vi "SHT41-string-array-to-data.vi"(9 "Starting Index":i32, 11 "Data In (string array)":string[](array[string])) -> (0 "SHT41: data output":T1 {"Humidity (%)" format="%.2f"; "Temp (degC)" format="%.2f"}, 2 "SHT41: Humidity (%)":dbl format="%.2f", 3 "SHT41: Temp (degC)":dbl format="%.2f")   [LabVIEW 2021]
uses:
  SHT41.ctl
panel:
  out "SHT41: Humidity":string
  out "SHT41: Temperature":string
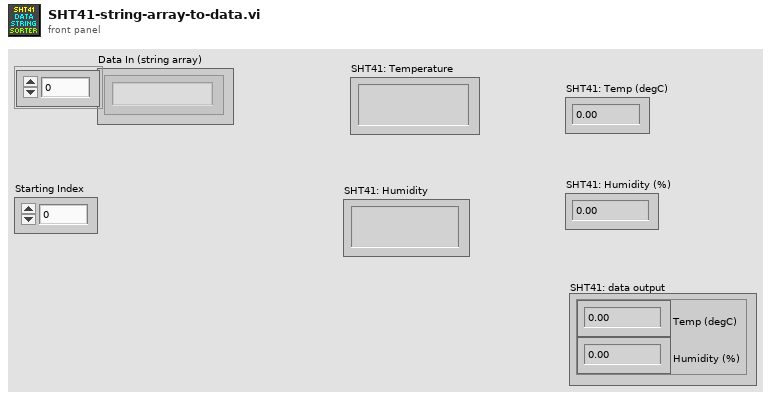
[diagram p1: front panel]
types:
  T1 = typedef "SHT41.ctl" = cluster{"Temp (degC)":dbl, "Humidity (%)":dbl}
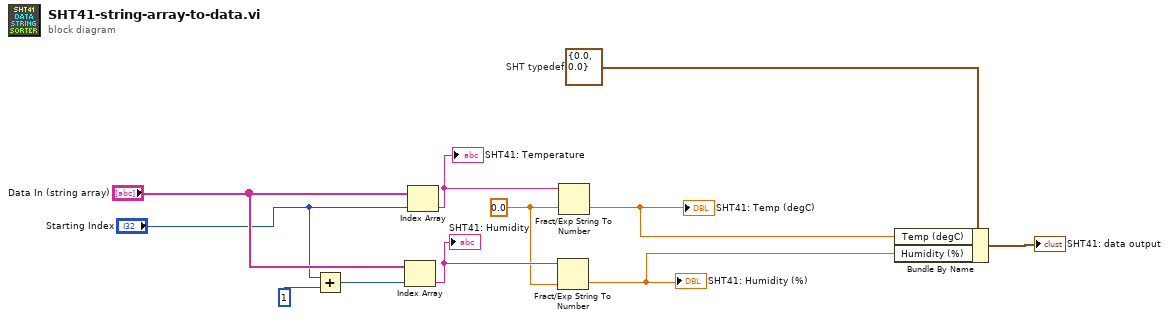
[diagram p0: block diagram]
diagram:
  w4 = T1 {"Temp (degC)"=0.0, "Humidity (%)"=0.0}  # SHT typedef
  w5 = 0.0
  n1 = Add(x="Starting Index", y=1) -> (x+y=w9:i32)
  n2 = Index Array(array="Data In (string array)", index=w9) -> (element=w6:string)
  "SHT41: Humidity" <- w6
  n3 = Index Array "Index Array"(array="Data In (string array)", index="Starting Index") -> (element=w7:string)
  "SHT41: Temperature" <- w7
  n4 = Fract/Exp String To Number(string=w6, default (0 dbl)=w5) -> (number=w2:dbl)  [unwired: 2 in, 1 out]
  "SHT41: Humidity (%)" <- w2
  n5 = Fract/Exp String To Number(string=w7, default (0 dbl)=w5) -> (number=w3:dbl)  [unwired: 2 in, 1 out]
  "SHT41: Temp (degC)" <- w3
  n6 = Bundle By Name(cluster=w4, "Temp (degC)"=w3, "Humidity (%)"=w2) -> (→"SHT41: data output":T1)
